vi "CaptureHWSynced.vi"(0 "object in":refnum<class "Hamamatsu.lvclass">=refnum, 5 "error in (no error)":errorcluster) -> (14 "object out":refnum<class "Hamamatsu.lvclass">, 16 "AllFramesAvailable?":bool, 17 "Frame Index":i32, 18 "Frame Count":i32, 19 "error out":errorcluster)   [LabVIEW 2019, in "Hamamatsu.lvclass"]
uses:
  Hamamatsu.lvclass
  Hamamatsu.lvclass/Hamamatsu.ctl
panel:
  out "Frames Skipped!":bool
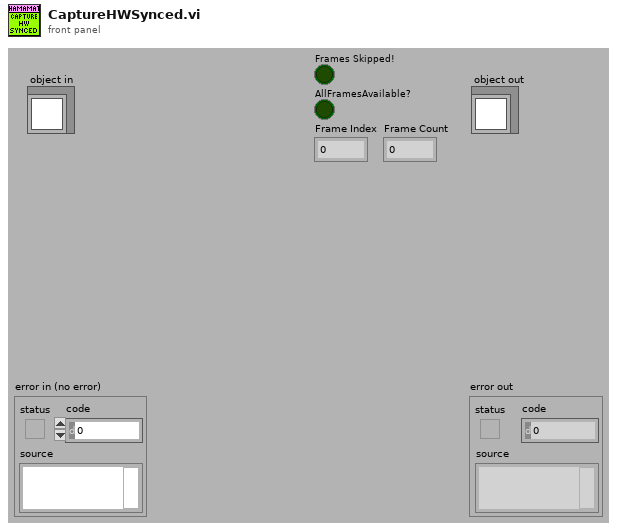
[diagram p1: front panel]
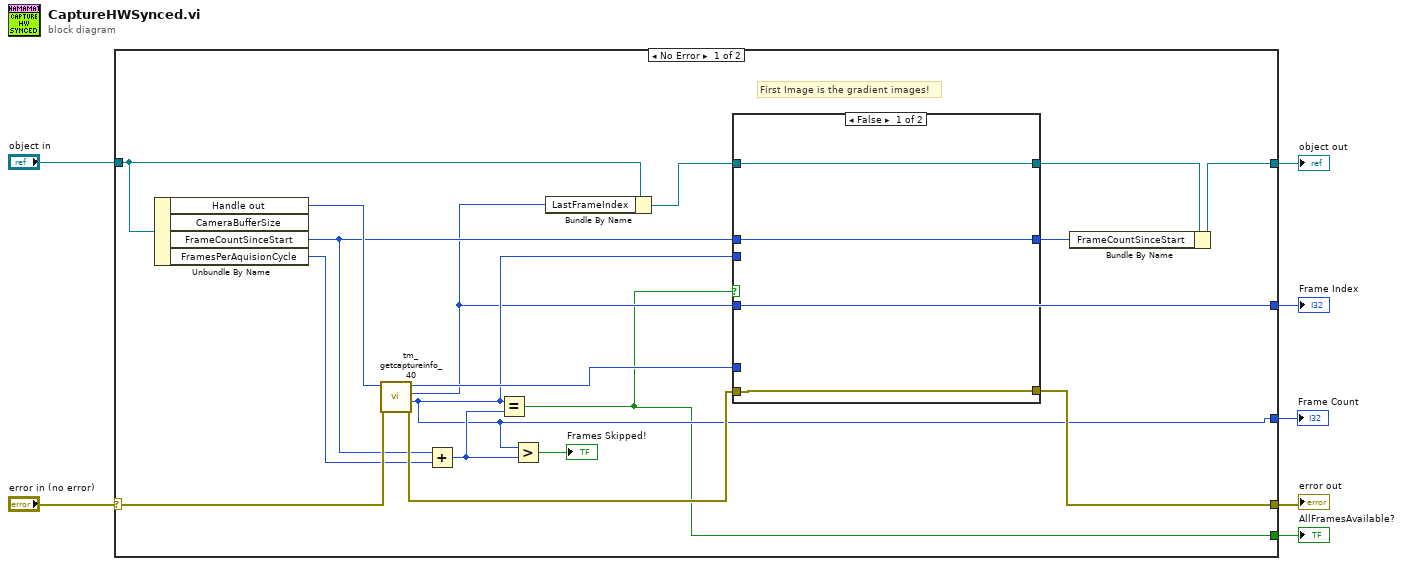
[diagram p0: block diagram]
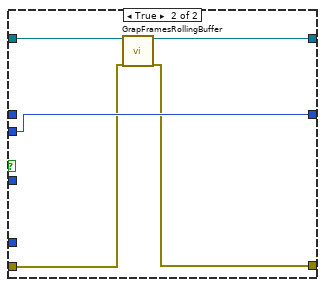
[diagram p2: hidden frame]
diagram:
  n1 = case shown="No Error" "error in (no error)" {
    selector: "error in (no error)" -> [w20 w34]
    tunnel: [w23 w34] -> w6
    tunnel: [w24 w33] -> w4
    tunnel: "object in" -> [w9 w33]
    tunnel: [w13 _] -> w3
    tunnel: [w12 _] -> w2
    tunnel: [w8 _] -> w1
    frame No Error {
      # "First Image is the gradient images!"
      n2 = Unbundle By Name(w9) -> ("Handle out"=w22:u32, "FrameCountSinceStart"=w14:i32, "FramesPerAquisionCycle"=w18:i32)  [unwired: 1 out]
      n3 = call <userlib>:"tm_getcaptureinfo_40.vi"("error in (no error)"=w20, "Handle in"=w22) -> ("error out"=w19:errorcluster, "Frame Count"=w13:i32, "Frame Index"=w12:i32, "Handle out"=w21:u32)  [unwired: 6 in]
      n4 = Add(x=w14, y=w18) -> (x+y=w17:i32)
      n5 = Equal?(x=w13, y=w17) -> (x = y?=w8:bool)
      n6 = Greater?(x=w13, y=w17) -> (0:→"Frames Skipped!":bool)
      n7 = Bundle By Name(cluster=w9, "LastFrameIndex"=w12) -> (w10:refnum<class "Hamamatsu.lvclass">)
      n8 = case shown="False" w8 {
        tunnel: [w26 w28] -> w23
        tunnel: w21 -> [_ _]
        tunnel: w19 -> [w26 w29]
        tunnel: [w27 w32] -> w15
        tunnel: w14 -> [w27 _]
        tunnel: w13 -> [_ w32]
        tunnel: w12 -> [_ _]
        tunnel: w10 -> [w25 w30]
        tunnel: [w25 w31] -> w11
        frame False {
        }
        frame True {
          n9 = call-dynamic "GrapFramesRollingBuffer.vi"("object in"=w30, "error in (no error)"=w29) -> ("object out"=w31:refnum<class "Hamamatsu.lvclass">, "error out"=w28:errorcluster)  [unwired: 16 in]
        }
      }
      n10 = Bundle By Name(cluster=w11, "FrameCountSinceStart"=w15) -> (w24:refnum<class "Hamamatsu.lvclass">)
    }
    frame Error {
    }
  }
  "error out" <- w6
  "object out" <- w4
  "Frame Index" <- w2
  "Frame Count" <- w3
  "AllFramesAvailable?" <- w1
